vi "booleanToString.vi"(11 "Boolean":bool=TRUE) -> (3 "String":string)   [LabVIEW 2011]
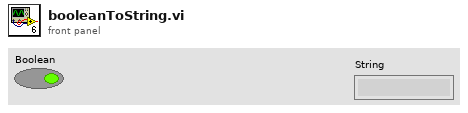
[diagram p1: front panel]
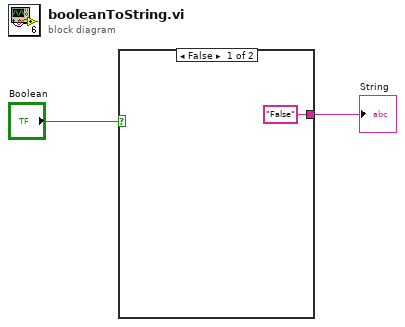
[diagram p0: block diagram]
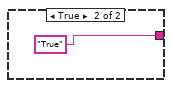
[diagram p2: hidden frame]
diagram:
  n1 = case shown="False" "Boolean" {
    tunnel: ["False" ("String") "True" ("String")] -> w1
    frame False {
    }
    frame True {
    }
  }
  "String" <- w1
